vi "Open existing emibin for reading.vi"(0 "file path":path, 11 "error in (no error)":errorcluster) -> (3 "File complete ID":u32, 4 "refnum out":refnum<file>, 6 "File type Std":u8 format="%.0x", 8 "File type ID":u16=1 format="%.0x", 10 "File type Version":u8 format="%.0x", 13 "size (in bytes)":i64, 14 "emibin OK":bool, 15 "error out":errorcluster)   [LabVIEW 2011]
uses:
  Header.ctl
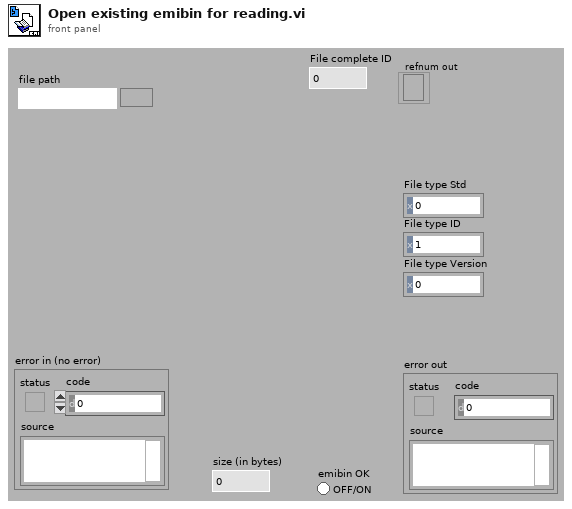
[diagram p1: front panel]
types:
  T1 = typedef "Header.ctl" = cluster{"Fixed code":u32, "File type Std":u8, "File type ID":u16, "File type Version":u8}
  T2 = enum16{"big-endian, network order", "native, host order", "little-endian"}
  T3 = enum16{"open", "replace", "create", "open or create", "replace or create", "replace or create with confirmation"}
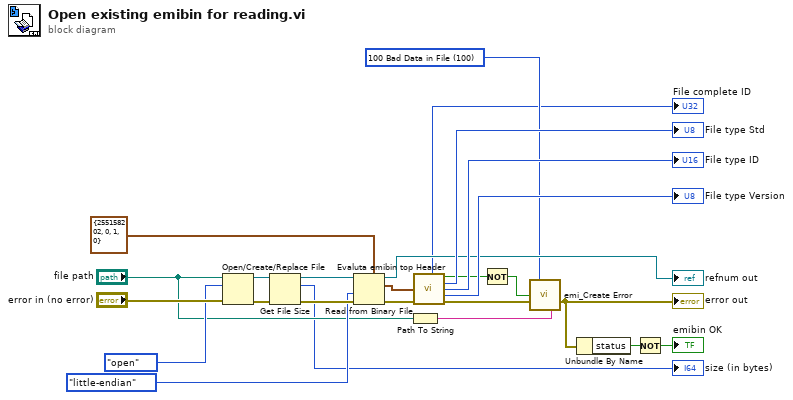
[diagram p0: block diagram]
diagram:
  w11 = 100 items=["0 No Error"=0, "1 Invalid input parameter"=1, "6 Generic file IO "=6, "7 File not Found"=7, "35 Generic Pring Error"=35, "37 Device not Found"=37, "39 Device Unit Error"=39, "40 Could fot Open Device"=40, "42 Generic Error"=42, "52 Unknown Message"=52, "98 Bad File type"=98, "99 Bad File Version"=99, "100 Bad Data in File"=100, "1018 Unspecefied Error"=1018, "1041 Incorrect Password"=1041, "1043 Feature not in this version"=1043, "1109 Unsuported Data type"=1109, "1444 Did not close sucessfully"=1444] ("Error Code")
  n1 = Open/Create/Replace File(file path (use dialog)="file path", error in="error in (no error)", operation (0:open)=T3."open") -> (refnum out=w22:refnum<file>, error out=w23:errorcluster)  [unwired: 3 in, 1 out]
  n2 = Get File Size(file=w22, error in=w23) -> (refnum out=w20:refnum<file>, size (in bytes)=→"size (in bytes)":i64, 0:w21:errorcluster)
  n3 = Read from Binary File(5:T1 {"Fixed code"=255158202, "File type Std"=0, "File type ID"=1, "File type Version"=0} ("bin ID header"), 8:w21, 9:T2."little-endian" ("byte order (0:big-endian, network order)"), 11:w20) -> (0:w17:errorcluster, 2:w16:T1, 3:→"refnum out":refnum<file>)  [unwired: 2 in, 1 out]
  n4 = Path To String(path="file path") -> (string=w7:string)
  n5 = call "Evaluta emibin top Header.vi"("bin ID header"=w16, "error in (no error)"=w17) -> ("File complete ID"=→"File complete ID":u32, "Correct Hader"=w9:bool, "File type Std"=→"File type Std":u8, "File type ID"=→"File type ID":u16, "File type Version"=→"File type Version":u8, "error out"=w10:errorcluster)  [unwired: 8 in]
  n6 = Not(x=w9) -> (.not. x?=w1:bool)
  n7 = call "emi_Create Error.vi"("Error Code"=w11, "Error(T)"=w1, "error in (no error)"=w10, "Append String(\"\")"=w7) -> ("error out"=w5:errorcluster)  [unwired: 11 in]
  "error out" <- w5
  n8 = Unbundle By Name(w5) -> ("status"=w4:bool)
  n9 = Not(x=w4) -> (.not. x?=→"emibin OK":bool)
